vi "Vision Research Phantom Series PhFile PhWriteCineFileAsync.vi"(0 "CH [in]":u64, 1 "pfnCallback [in]":u32, 5 "Error In (no error)":errorcluster) -> (14 "CH [out]":u64, 15 "pfnCallback [out]":u32, 19 "Error Out":errorcluster)   [LabVIEW 2013, in "VRI.lvlib"]
doc: "PhWriteCineFileAsync\nHRESULT PhWriteCineFileAsync(CINEHANDLE CH, PROGRESSCB pfnCallback);\n\nParameters\nCH [in]\n Cine to be saved.\npfnCallback [in, optional]\n Pointer to the progress callback function which shows the amount of work done.\n It can be NULL.\n\nReturn Value\nThe function returns ERR_Ok in case of success or an error code, otherwise. To get extended error information call PhGetErrorMessage.\n\nRemarks\nAsynchronous function used for saving a cine to file.\nAsynchronous equivalent of PhWriteCineFile.\nIt starts a thread responsible for writing the file and immediately returns.\nWhen the write operation finishes either because an error was encountered or because all data has been written to file, the callback function is called with the percent parameter set to 100.\nTo differentiate between the two possible situations, the caller should call PhGetCineInfo with GCI_WRITEERR code selector to check if any error was encountered.\nAt most one save operation per cine can be active at any given time.\nCall PhStopWriteCineFileAsync to abort an asynchronous save operation.\n\nRequired Header\nPhFile.h"
uses:
  VRI.lvlib
  Phantom DLLs/PhFile.dll
panel:
  # "For instructions on the use of this VI, press Ctrl+H to display the help window and move the mouse over the icon, controls, and indicators"
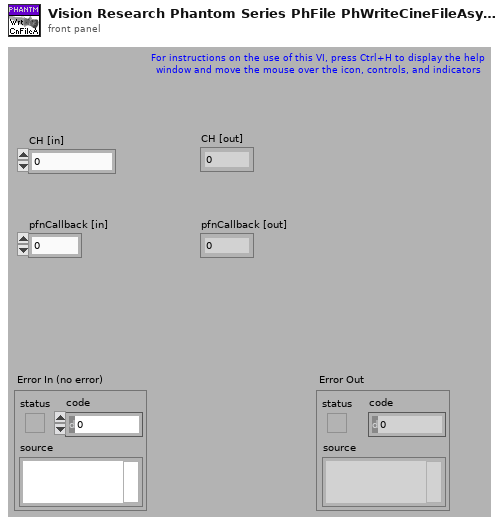
[diagram p1: front panel]
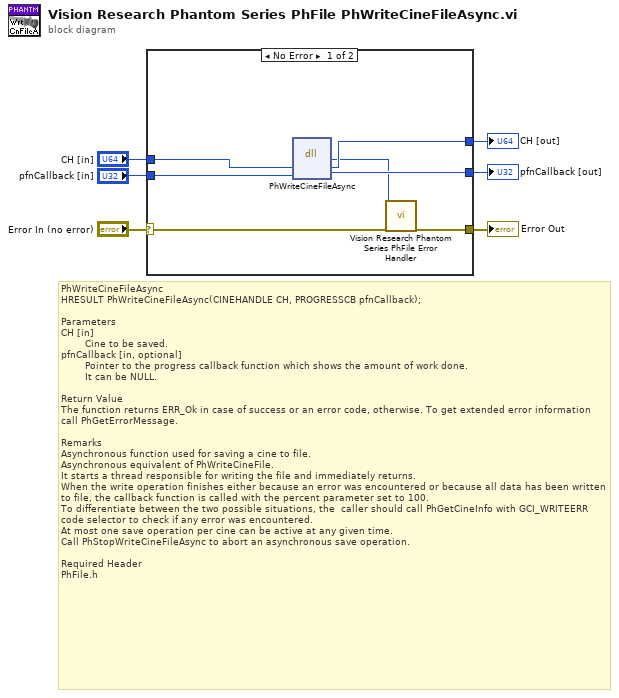
[diagram p0: block diagram]
diagram:
  # "PhWriteCineFileAsync\nHRESULT PhWriteCineFileAsync(CINEHANDLE CH, PROGRESSCB pfnCallback);\n\nParameters\nCH [in]\n        Cine to be saved.\npfnCallback [in, optional]\n        Pointer to the progress callback function which shows the amount of work done.\n       \tIt can be NULL.\n\nReturn Value\nThe function returns ERR_Ok in case of success or an error code, otherwise. To get extended error information call PhGetErrorMessage.\n\nRemarks\nAsynchronous function used for saving a cine to file.\nAsynchronous equivalent of PhWriteCineFile.\nIt starts a thread responsible for writing the file and immediately returns.\nWhen the write operation finishes either because an error was encountered or because all data has been written to file, the callback function is called with the percent parameter set to 100.\nTo differentiate between the two possible situations, the \tcaller should call PhGetCineInfo with GCI_WRITEERR code selector to check if any error was encountered.\nAt most one save operation per cine can be active at any given time.\nCall PhStopWriteCineFileAsync to abort an asynchronous save operation.\n\nRequired Header\nPhFile.h"
  n1 = case shown="No Error" "Error In (no error)" {
    selector: "Error In (no error)" -> [w13 w16]
    tunnel: [w12 w16] -> w5
    tunnel: "pfnCallback [in]" -> [w11 w15]
    tunnel: "CH [in]" -> [w10 w14]
    tunnel: [w9 w15] -> w2
    tunnel: [w8 w14] -> w1
    frame No Error {
      n2 = dll-call lib="C:/Projects/SDK/32-bit/Vision Research Phantom Series Labview Driver/Phantom DLLs/PhFile.dll" fn="PhWriteCineFileAsync"("CH"=w10, "pfnCallback"=w11) -> ("HRESULT"=w7:i32, "CH"=w8:u64, "pfnCallback"=w9:u32)  [unwired: 3 in, 2 out]
      n3 = call "Vision Research Phantom Series PhFile Error Handler.vi"("Error Code (0)"=w7, "Error In (no error)"=w13) -> ("Error Out"=w12:errorcluster)  [unwired: 17 out]
    }
    frame Error {
    }
  }
  "Error Out" <- w5
  "pfnCallback [out]" <- w2
  "CH [out]" <- w1
